vi "Include Parents.vi"(7 "Linker Tree Map":map{i32, i32}(c390), 11 "Tree":T1[](array[typedef])) -> (3 "Updated Tree":T1[](array[typedef]))   [LabVIEW 2020, in "Linker Info.lvlib"]
uses:
  Linker Info.lvlib
  Tree Item.ctl
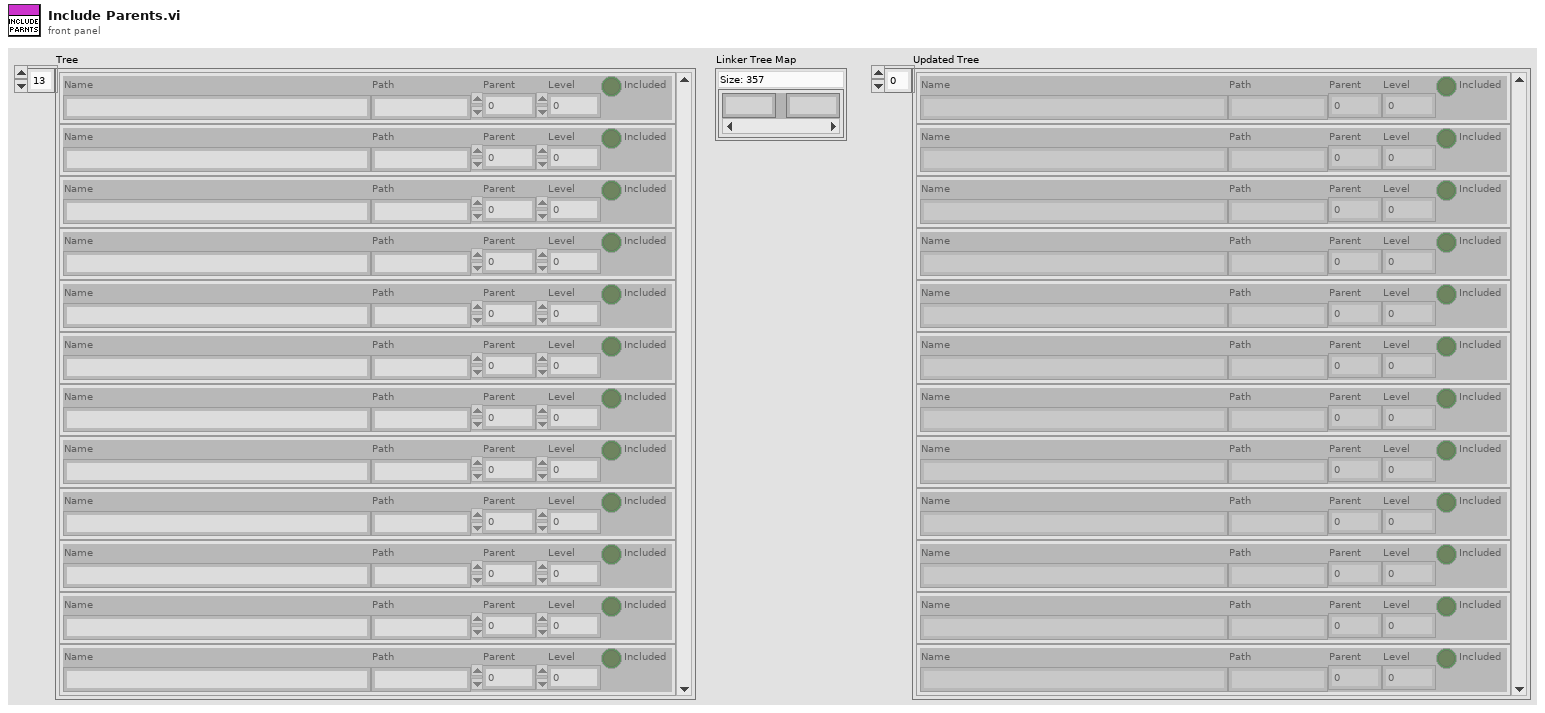
[diagram p1: front panel]
types:
  T1 = typedef "Linker Info.lvlib/Tree Item.ctl" = cluster{"Name":string, "Path":string, "Parent":i32, "Level":i32, "Included":bool}
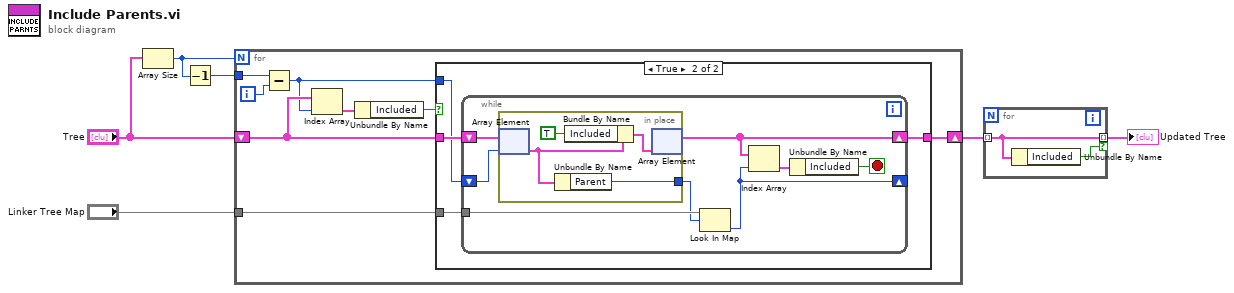
[diagram p0: block diagram]
diagram:
  n1 = Array Size(array="Tree") -> (size(s)=w5:i32)
  n2 = Decrement(x=w5) -> (x-1=w4:i32)
  n3 = for {
    N: w5 -> [_]
    shift-right: [w8] -> w2
    shift-left: "Tree" -> [w11]
    tunnel: w4 -> [w14]
    tunnel: "Linker Tree Map" -> [w7]
    i -> [w13]
    n4 = Subtract(x=w14, y=w13) -> (x-y=w9:i32)
    n5 = Index Array(array=w11, index=w9) -> (element=w12:T1)
    n6 = Unbundle By Name(w12) -> ("Included"=w10:bool)
    n7 = case shown="True" w10 {
      tunnel: w11 -> [w15 w19]
      tunnel: w9 -> [_ w18]
      tunnel: [w15 w17] -> w8
      tunnel: w7 -> [_ w16]
      frame False {
      }
      frame True {
        n8 = while {
          shift-right: [w25] -> w17
          shift-left: w19 -> [w27]
          shift-right: [w20] -> _
          shift-left: w18 -> [w26]
          tunnel: w16 -> [w22]
          stop <- w23 stop-if-true
          n9 = in-place {
            in-place-border: [w28] -> w21
            n10 = in-place-array #1(w27, w26) -> (w31:T1)
            n11 = Unbundle By Name(w31) -> ("Parent"=w28:i32)
            n12 = Bundle By Name(cluster=w31, "Included"=TRUE) -> (w29:T1)
            n13 = in-place-array #1(w29) -> (w25:T1[])  [unwired: 1 out]
          }
          n14 = Look In Map(map=w22, key=w21) -> (value=w20:i32)  [unwired: 1 in, 1 out]
          n15 = Index Array(array=w25, index=w20) -> (element=w24:T1)
          n16 = Unbundle By Name(w24) -> ("Included"=w23:bool)
        }
      }
    }
  }
  n17 = for {
    tunnel: w2 -> [w33] mode=indexing
    tunnel: [w33] -> w1 mode=indexing if=w32
    n18 = Unbundle By Name(w33) -> ("Included"=w32:bool)
  }
  "Updated Tree" <- w1
